vi "calculate_histogram.vi"(8 "error in (no error)":errorcluster, 9 "# bins [100]":i32=100, 10 "# std deviations for histogram width [1]":dbl=1.0, 11 "Intensity Graph":dbl[][](array[numeric])) -> (0 "error out":errorcluster, 1 "standard deviation":dbl format="%0.2f", 2 "mean":dbl format="%0.2f", 3 "Histogram Graph":T1(graph))   [LabVIEW 2019, in "graph_utilities.lvclass"]
uses:
  graph_utilities.lvclass
  <vilib>/Analysis/NI_AALPro.lvlib
  <vilib>/Analysis/NI_AALBase.lvlib
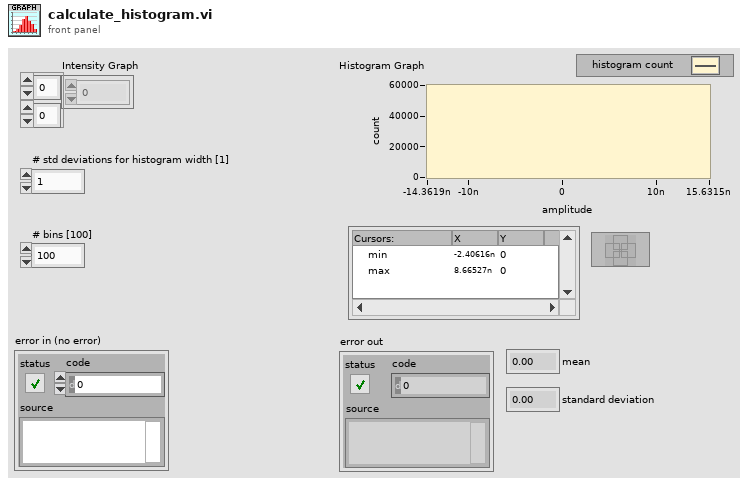
[diagram p1: front panel]
types:
  T1 = cluster{"X Values":dbl[], "Histogram: h(x)":i32[]}
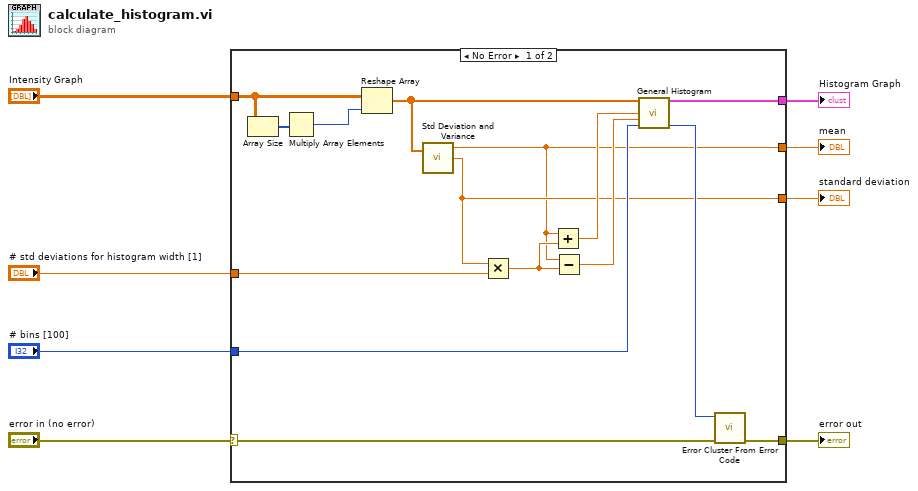
[diagram p0: block diagram]
diagram:
  n1 = case shown="No Error" "error in (no error)" {
    selector: "error in (no error)" -> [w15 w24]
    tunnel: "# std deviations for histogram width [1]" -> [w21 _]
    tunnel: "# bins [100]" -> [w19 _]
    tunnel: [w18 _] -> w6
    tunnel: "Intensity Graph" -> [w9 _]
    tunnel: [w14 w24] -> w3
    tunnel: [w13 _] -> w2
    tunnel: [w12 _] -> w1
    frame No Error {
      n2 = Array Size(array=w9) -> (size(s)=w11:i32[])
      n3 = Multiply Array Elements(1:w11) -> (0:w10:i32)
      n4 = Reshape Array(w9, w10) -> (w17:dbl[])
      n5 = call <vilib>:"Std Deviation and Variance.vi"("X"=w17) -> ("mean"=w12:dbl, "standard deviation"=w13:dbl)  [unwired: 1 in, 1 out]
      n6 = Multiply(x=w13, y=w21) -> (x*y=w20:dbl)
      n7 = Add(x=w12, y=w20) -> (x+y=w23:dbl)
      n8 = Subtract(x=w12, y=w20) -> (x-y=w22:dbl)
      n9 = call <vilib>:"General Histogram.vi"("X"=w17, "max"=w23, "min"=w22, "# bins"=w19) -> ("Histogram Graph"=w18:T1, "error"=w16:i32)  [unwired: 7 in, 3 out]
      n10 = call <vilib>:"Error Cluster From Error Code.vi"("error in (no error)"=w15, "error code (0)"=w16) -> ("error out"=w14:errorcluster)  [unwired: 7 in]
    }
    frame Error {
    }
  }
  "Histogram Graph" <- w6
  "error out" <- w3
  "standard deviation" <- w2
  "mean" <- w1
